vi "PING logger.vi"() -> ()   [LabVIEW 2013]
panel:
  out "record ON":bool
  in  "Autoscale":bool=TRUE
  in  "send ping each [ms]":u32=500
  in  "Exit":bool
  in  "Record":bool
  out "XY Graph 2":cluster{timestamp[], i32[]}(graph)
  in  "Stop capture":bool
  out "actual ping time":i32
  out "CMD output":string
  in  "command line":string="ping www.vutbr.cz -n 1"
  # "PING TIME LOGGER"
  # "note: -1 value means error"
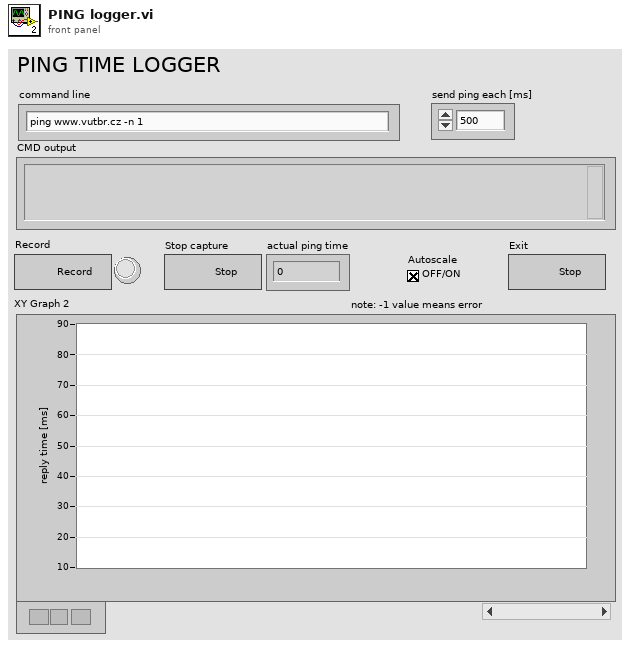
[diagram p1: front panel]
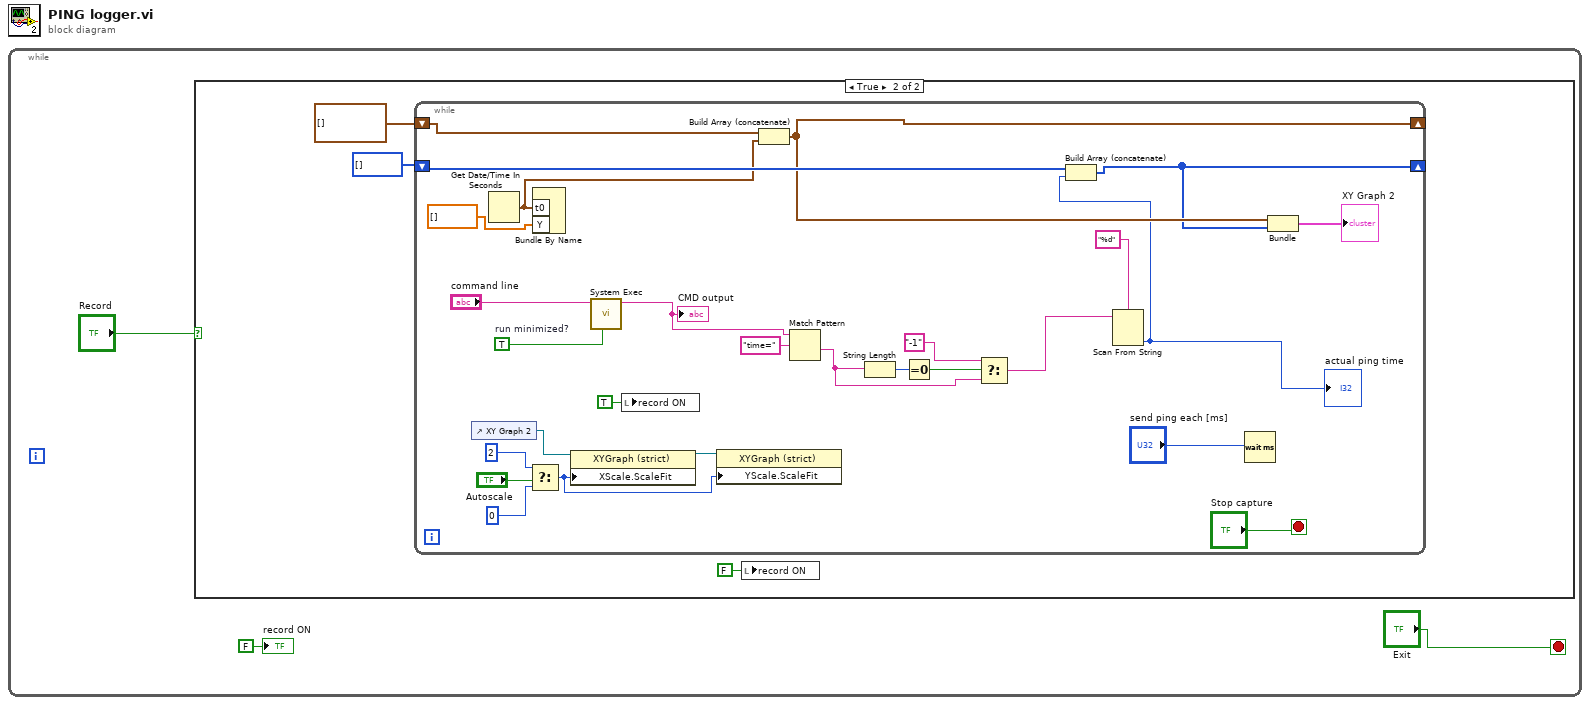
[diagram p0: block diagram]
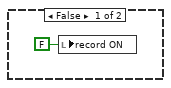
[diagram p2: hidden frame]
diagram:
  n1 = while {
    stop <- "Exit" stop-if-true
    n2 = case shown="True" "Record" {
      frame False {
        n3 = local write "record ON"(FALSE ("record ON")) -> ()
      }
      frame True {
        n4 = while {
          shift-right: [w27] -> _
          shift-left: i32[] [] -> [w32]
          shift-right: [w28] -> _
          shift-left: timestamp[] [] -> [w29]
          stop <- "Stop capture" stop-if-true
          w22 = TRUE  # run minimized?
          n5 = control-ref of="XY Graph 2"() -> (w10:refnum<vi>)
          n6 = Get Date/Time In Seconds() -> (seconds since 1Jan1904=w24:timestamp)
          n7 = Select(t=u8 2 ("X Scale.Scale Fit"), s="Autoscale", f=u8 0 ("X Scale.Scale Fit")) -> (s? t:f=w13:u8)
          n8 = Bundle By Name("t0"=w24, "Y"=dbl[] []) -> ()  [unwired: 1 in, 1 out]
          n9 = property on="Property Node" class="XYGraph (strict)"(reference=w10, "XScale.ScaleFit"=w13) -> ()  [unwired: 1 in, 2 out]
          n10 = call <vilib>:"System Exec.vi"("run minimized? (F)"=w22, "command line"="command line") -> ("standard output"=w20:string)  [unwired: 4 in, 5 out]
          "CMD output" <- w20
          n11 = local write "record ON"(TRUE ("record ON")) -> ()
          n12 = property on="Property Node" class="XYGraph (strict)"(reference=w10, "YScale.ScaleFit"=w13) -> ()  [unwired: 1 in, 2 out]
          n13 = Build Array (concatenate)(w29, w24) -> (w28:timestamp[])
          n14 = Match Pattern(string=w20, regular expression="time=") -> (after substring=w16:string)  [unwired: 1 in, 3 out]
          n15 = String Length(string=w16) -> (length=w19:i32)
          n16 = Equal To 0?(x=w19) -> (x = 0?=w18:bool)
          n17 = Select(t="-1" ("regular expression"), s=w18, f=w16) -> (s? t:f=w15:string)
          n18 = Scan From String(format string="%d", input string=w15) -> (output 1=w14:i32)  [unwired: 3 in, 3 out]
          "actual ping time" <- w14
          n19 = Build Array (concatenate)(w32, w14) -> (w27:i32[])
          n20 = Wait (ms)(milliseconds to wait="send ping each [ms]") -> ()  [unwired: 1 out]
          n21 = Bundle(w28, w27) -> (→"XY Graph 2":cluster{timestamp[], i32[]})  [unwired: 1 in]
        }
        n22 = local write "record ON"(FALSE ("record ON")) -> ()
      }
    }
    "record ON" <- FALSE ("record ON")
  }
